vi "Begin.vi"(11 "Image Size":T1=enum."320x240") -> (0 "error out":errorcluster)   [LabVIEW 2012]
doc: "Called before other user functions, this VI is expected to open initial I/O refnums, load in file data, and do all program initialization. Notice that the <B>error out</B> terminal is simply used for data flow. Wiring it to other structures or subVIs ensures that this VI runs first."
uses:
  <vilib>/Rock Robotics/WPI/Camera/WPI_CameraImageSize.ctl
  <vilib>/Rock Robotics/WPI/DriverStation/WPI_DriverStationRobotMode2.ctl
  <vilib>/Rock Robotics/SystemInterfaces/DIO/FPGA_DIOPWMChannel.ctl
  <vilib>/Rock Robotics/WPI/Joystick/WPI_JoystickDeviceEnum.ctl
  <vilib>/Rock Robotics/WPI/Relay/WPI_RelayDirection.ctl
  <vilib>/Rock Robotics/SystemInterfaces/DIO/FPGA_DIORelayChannel.ctl
  <vilib>/Rock Robotics/SystemInterfaces/AI/FPGA_AIChannel.ctl
  <vilib>/Rock Robotics/SystemInterfaces/AI/FPGA_AIGyroChannel.ctl
  <vilib>/Rock Robotics/SystemInterfaces/DIO/FPGA_DIOChannel.ctl
  <vilib>/Rock Robotics/SystemInterfaces/Typedef/FPGA_TypedefDigitalModule.ctl
  Robot Global Data.vi
  <vilib>/Rock Robotics/WPI/MotorControl/WPI_MotorControlOpen Victor.vi
  <vilib>/Rock Robotics/WPI/Camera/WPI_CameraFrameRate.ctl
panel:
  in  "Input":dbl
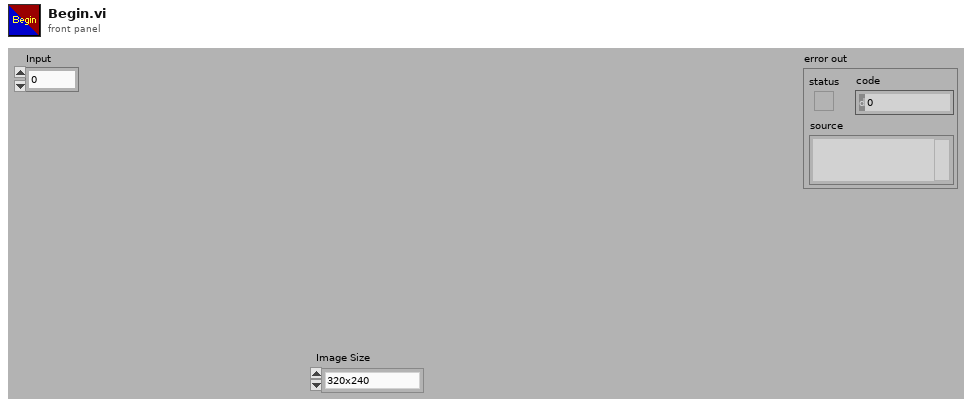
[diagram p1: front panel]
types:
  T1 = typedef "WPI_CameraImageSize.ctl" = enum16{"640x480", "320x240", "160x120"}
  T2 = typedef "FPGA_DIOChannel.ctl" = enum8{"DIO 1", "DIO 2", "DIO 3", "DIO 4", "DIO 5", "DIO 6", "DIO 7", "DIO 8", "DIO 9", "DIO 10", "DIO 11", "DIO 12", "DIO 13", "DIO 14", "Invalid"}
  T3 = typedef "FPGA_TypedefDigitalModule.ctl" = enum16{"Digital Module 1", "Digital Module 2"}
  T4 = typedef "FPGA_DIOPWMChannel.ctl" = enum8{"PWM 1", "PWM 2", "PWM 3", "PWM 4", "PWM 5", "PWM 6", "PWM 7", "PWM 8", "PWM 9", "PWM 10", "Invalid"}
  T5 = typedef "FPGA_DIORelayChannel.ctl" = enum8{"Relay 1", "Relay 2", "Relay 3", "Relay 4", "Relay 5", "Relay 6", "Relay 7", "Relay 8", "Invalid"}
  T6 = typedef "WPI_RelayDirection.ctl" = enum16{"Both directions", "Forward only", "Reverse only"}
  T7 = typedef "FPGA_AIChannel.ctl" = enum8{"AI 1", "AI 2", "AI 3", "AI 4", "AI 5", "AI 6", "AI 7", "AI 8", "Invalid"}
  T8 = typedef "FPGA_AIGyroChannel.ctl" = enum8{"AI 1", "AI 2", "Invalid"}
  T9 = typedef "WPI_JoystickDeviceEnum.ctl" = enum16{"USB 1", "USB 2", "USB 3", "USB 4", "Kinect 1", "Kinect 2"}
  T10 = typedef "WPI_DriverStationRobotMode2.ctl" = enum16{"Autonomous Disabled", "Autonomous Enabled", "Teleop Disabled", "Teleop Enabled", "Timeout", "Finish", "Test Disabled", "Test Enabled"}
  T11 = typedef "WPI_RelayDevRef.ctl" = cluster{"DevStatus":errorcluster, "Relay Channel":T5, "Digital Module":T3, "Relay Direction":T6}
  T12 = typedef "WPI_CameraFrameRate.ctl" = u32
  T13 = typedef "WPI_CameraDevRef.ctl" = cluster{"Camera Address":string, "CameraStatus":errorcluster, "Acquire Image Notifier":refnum<notifier>}
  T14 = typedef "WPI_MotorControlDeviceRef.ctl" = cluster{"DeviceStatus":errorcluster, "Type":enum16{"PWM", "CAN"}, "PWM":cluster{"Digital Module":T3, "PWM Channel":T4, "DeadBand":T15}, "CAN":cluster{"Device Number":u8, "Control Mode":T16, "Semaphore":T17, "Max Vout":dbl}, "Invert":bool, "TransformRef":T18, "InvTransformRef":T18}
  T15 = typedef "WPI_PWMDeadband.ctl" = cluster{"Name":string, "maxPositivePwm":i32, "minPositivePwm":i32, "centerPwm":i32, "maxNegativePwm":i32, "minNegativePwm":i32, "angularRange":u16}
  T16 = typedef "WPI_CANJaguar_ControlMode.ctl" = enum8{"Percent VBus", "Current", "Speed", "Position", "Voltage"}
  T17 = typedef "Semaphore RefNum" = refnum<k1>
  T18 = typedef "WPI_PWMTransform_ConPane.ctl" = refnum<vi>
  T19 = typedef "WPI_JoystickDevRef.ctl" = cluster{"Device":T9}
  T20 = typedef "WPI_ServoDeviceRef.ctl" = cluster{"DeviceStatus":errorcluster, "Digital Module":T3, "PWM Channel":T4, "DeadBand":T15}
  T21 = cluster{"Setpoint 1":dbl, "Setpoint 2":dbl, "Setpoint 3":dbl, "Setpoint 4":dbl, "RotLow":dbl, "RotHigh":dbl, "ExtLow":dbl, "ExtHigh":dbl}
  T22 = typedef "WPI_DigitalInputDevRef.ctl" = cluster{"DevStatus":errorcluster, "DIO Channel":T2, "Digital Module":T3}
  T23 = typedef "WPI_AnalogChannelDevRef.ctl" = cluster{"DevStatus":errorcluster, "Analog Module":T24, "Analog Channel":T7}
  T24 = typedef "FPGA_TypedefAnalogModule.ctl" = enum16{"Analog Module 1", "Analog Module 2"}
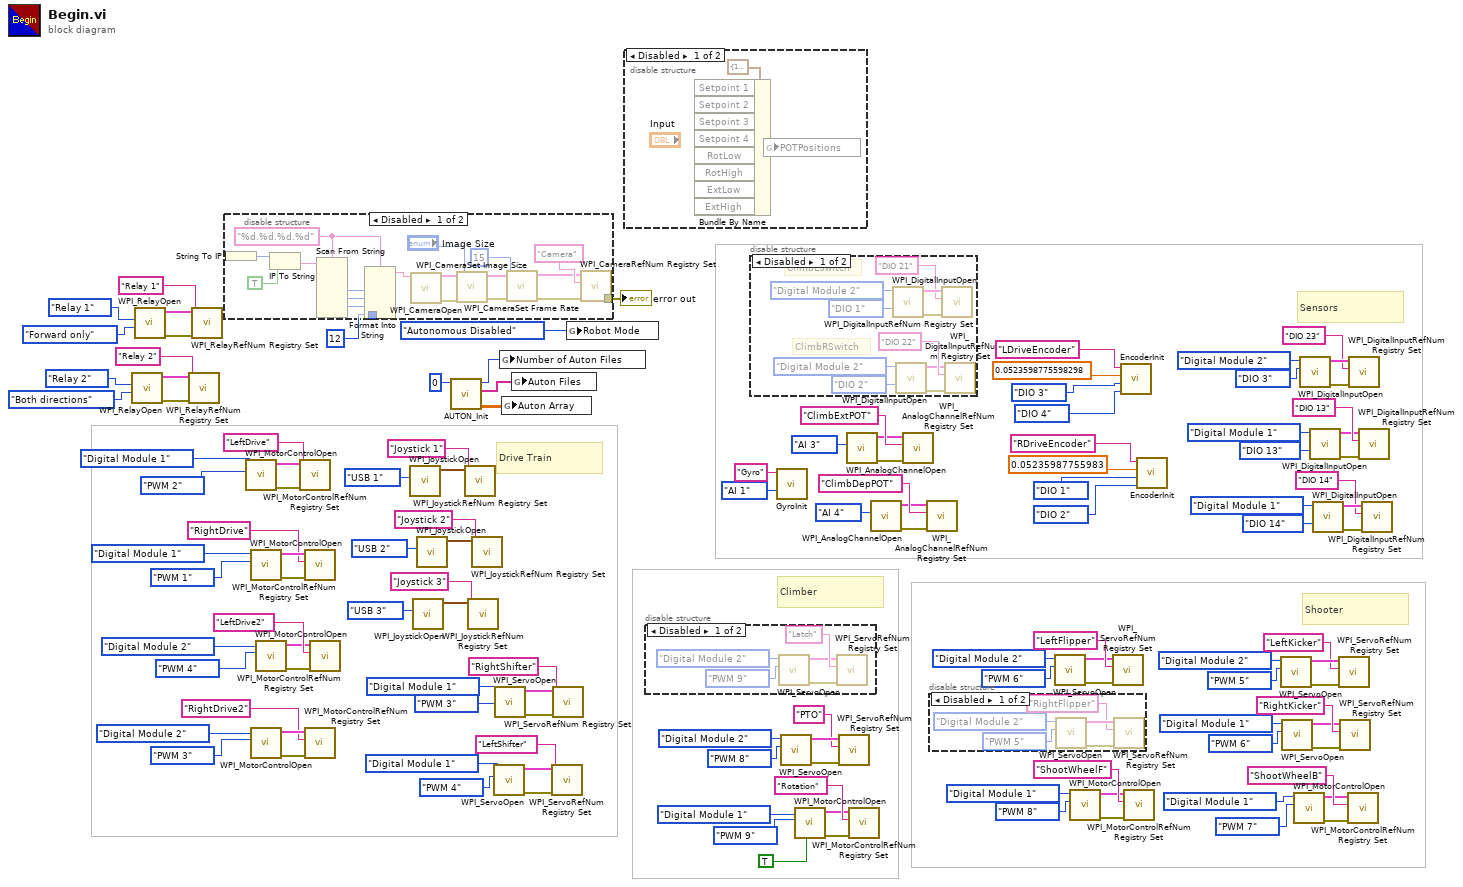
[diagram p0: block diagram]
diagram:
  # "Shooter"
  # "Drive Train"
  # "Climber"
  # "Sensors"
  n1 = call <vilib>:"WPI_RelayOpen.vi"("Relay Direction"=WPI_RelayDirection."Both directions", "Relay Channel"=FPGA_DIORelayChannel."Relay 2") -> ("error out"=w87:errorcluster, "RelayDevRef"=w88:T11)  [unwired: 8 in]
  n2 = call <vilib>:"WPI_RelayOpen.vi"("Relay Direction"=WPI_RelayDirection."Forward only", "Relay Channel"=FPGA_DIORelayChannel."Relay 1") -> ("error out"=w45:errorcluster, "RelayDevRef"=w44:T11)  [unwired: 8 in]
  n3 = call <vilib>:"WPI_RelayRefNum Registry Set.vi"("error in (no error)"=w87, "refnum name"="Relay 2", "RelayDevRef"=w88) -> ()  [unwired: 7 in, 2 out]
  n4 = call <vilib>:"WPI_RelayRefNum Registry Set.vi"("error in (no error)"=w45, "refnum name"="Relay 1", "RelayDevRef"=w44) -> ()  [unwired: 7 in, 2 out]
  n5 = disable-structure shown="Disabled" {
    disable-tunnel: 12 ("Compression") -> [w136 _]
    disable-tunnel: [w126 _] -> w46
    frame Disabled {
      w135 = "%d.%d.%d.%d" ("format string")
      n6 = String To IP() -> (0:w142:u32)  [unwired: 1 in]
      n7 = IP To String(1:TRUE ("dot notation? (F)"), 2:w142) -> (0:w140:string)
      n8 = Scan From String(format string=w135, input string=w140) -> (output 1=w139:i32, output 2=w138:i32, output 3=w137:i32)  [unwired: 7 in, 3 out]
      n9 = Format Into String(format string=w135, w139, w138, w137, w136) -> (resulting string=w134:string)  [unwired: 2 in, 1 out]
      n10 = call <vilib>:"WPI_CameraOpen.vi"("Camera Address"=w134) -> ("error out"=w133:errorcluster, "CameraDevRef"=w132:T13)  [unwired: 1 in, 8 out]
      n11 = call <vilib>:"WPI_CameraSet Image Size.vi"("error in (no error)"=w133, "Image Size"="Image Size", "CameraDevRef"=w132) -> ("error out"=w130:errorcluster, "CameraDevRef Out"=w131:T13)  [unwired: 7 out]
      n12 = call <vilib>:"WPI_CameraSet Frame Rate.vi"("error in (no error)"=w130, "Frame Rate (fps)"=T12 15, "CameraDevRef"=w131) -> ("error out"=w129:errorcluster, "CameraDevRef Out"=w128:T13)  [unwired: 7 out]
      n13 = call <vilib>:"WPI_CameraRefNum Registry Set.vi"("error in (no error)"=w129, "refnum name"="Camera", "CameraDevRef"=w128) -> ("error out"=w126:errorcluster)  [unwired: 8 out]
    }
    frame Enabled {
    }
  }
  "error out" <- w46
  n14 = call-poly <vilib>:"WPI_MotorControlOpen.vi"("PWM Channel"=FPGA_DIOPWMChannel."PWM 2", "Digital Module (Module 1)"=FPGA_TypedefDigitalModule."Digital Module 1") -> ("error out"=w113:errorcluster, "MotorControlDeviceRef"=w114:T14)  [unwired: 8 in]
  n15 = call-poly <vilib>:"WPI_MotorControlOpen.vi"("PWM Channel"=FPGA_DIOPWMChannel."PWM 1", "Digital Module (Module 1)"=FPGA_TypedefDigitalModule."Digital Module 1") -> ("error out"=w120:errorcluster, "MotorControlDeviceRef"=w119:T14)  [unwired: 8 in]
  n16 = call-poly <vilib>:"WPI_MotorControlOpen.vi"("PWM Channel"=FPGA_DIOPWMChannel."PWM 3", "Digital Module (Module 1)"=FPGA_TypedefDigitalModule."Digital Module 2") -> ("error out"=w102:errorcluster, "MotorControlDeviceRef"=w101:T14)  [unwired: 8 in]
  n17 = call-poly <vilib>:"WPI_MotorControlOpen.vi"("PWM Channel"=FPGA_DIOPWMChannel."PWM 4", "Digital Module (Module 1)"=FPGA_TypedefDigitalModule."Digital Module 2") -> ("error out"=w93:errorcluster, "MotorControlDeviceRef"=w94:T14)  [unwired: 8 in]
  n18 = call <vilib>:"WPI_MotorControlRefNum Registry Set.vi"("error in (no error)"=w113, "refnum name"="LeftDrive", "MotorControlDevRef"=w114) -> ()  [unwired: 7 in, 2 out]
  n19 = call <vilib>:"WPI_MotorControlRefNum Registry Set.vi"("error in (no error)"=w120, "refnum name"="RightDrive", "MotorControlDevRef"=w119) -> ()  [unwired: 7 in, 2 out]
  n20 = call <vilib>:"WPI_MotorControlRefNum Registry Set.vi"("error in (no error)"=w102, "refnum name"="RightDrive2", "MotorControlDevRef"=w101) -> ()  [unwired: 7 in, 2 out]
  n21 = call <vilib>:"WPI_MotorControlRefNum Registry Set.vi"("error in (no error)"=w93, "refnum name"="LeftDrive2", "MotorControlDevRef"=w94) -> ()  [unwired: 7 in, 2 out]
  n22 = call <vilib>:"WPI_JoystickOpen.vi"("JoystickDevice"=WPI_JoystickDeviceEnum."USB 1") -> ("JoystickDevRef"=w104:T19)  [unwired: 10 in]
  n23 = call <vilib>:"WPI_JoystickOpen.vi"("JoystickDevice"=WPI_JoystickDeviceEnum."USB 3") -> ("JoystickDevRef"=w110:T19)  [unwired: 10 in]
  n24 = call <vilib>:"WPI_JoystickOpen.vi"("JoystickDevice"=WPI_JoystickDeviceEnum."USB 2") -> ("JoystickDevRef"=w109:T19)  [unwired: 10 in]
  n25 = call "AUTON_Init.vi"("Default File"=0) -> ("Auton Array"=w121:dbl[][], "Auton Files"=w122:string[], "Number of Auton Files"=w123:i64)  [unwired: 8 in]
  n26 = call <vilib>:"WPI_JoystickRefNum Registry Set.vi"("refnum name"="Joystick 1", "JoystickDevRef"=w104) -> ()  [unwired: 8 in, 2 out]
  n27 = call <vilib>:"WPI_JoystickRefNum Registry Set.vi"("refnum name"="Joystick 3", "JoystickDevRef"=w110) -> ()  [unwired: 8 in, 2 out]
  n28 = call <vilib>:"WPI_JoystickRefNum Registry Set.vi"("refnum name"="Joystick 2", "JoystickDevRef"=w109) -> ()  [unwired: 8 in, 2 out]
  n29 = call <vilib>:"WPI_ServoOpen.vi"("PWM Channel"=FPGA_DIOPWMChannel."PWM 4", "Digital Module (Module 1)"=FPGA_TypedefDigitalModule."Digital Module 1") -> ("error out"=w86:errorcluster, "ServoDeviceRef"=w79:T20)  [unwired: 8 in]
  n30 = call <vilib>:"WPI_ServoOpen.vi"("PWM Channel"=FPGA_DIOPWMChannel."PWM 3", "Digital Module (Module 1)"=FPGA_TypedefDigitalModule."Digital Module 1") -> ("error out"=w85:errorcluster, "ServoDeviceRef"=w84:T20)  [unwired: 8 in]
  n31 = global write "Robot Global Data.vi" "Number of Auton Files"(w123) -> ()
  n32 = global write "Robot Global Data.vi" "Auton Array"(w121) -> ()
  n33 = global write "Robot Global Data.vi" "Auton Files"(w122) -> ()
  n34 = call <vilib>:"WPI_ServoRefNum Registry Set.vi"("error in (no error)"=w86, "refnum name"="LeftShifter", "ServoDeviceRef"=w79) -> ()  [unwired: 7 in, 2 out]
  n35 = call <vilib>:"WPI_ServoRefNum Registry Set.vi"("error in (no error)"=w85, "refnum name"="RightShifter", "ServoDeviceRef"=w84) -> ()  [unwired: 7 in, 2 out]
  n36 = global write "Robot Global Data.vi" "Robot Mode"(WPI_DriverStationRobotMode2."Autonomous Disabled" ("Robot Mode")) -> ()
  n37 = disable-structure shown="Disabled" {
    frame Disabled {
      n38 = Bundle By Name(cluster=T21 {"Setpoint 1"=1.95, "Setpoint 2"=2.1, "Setpoint 3"=2.2, "Setpoint 4"=2.25, "RotLow"=1.92, "RotHigh"=2.3, "ExtLow"=1.87, "ExtHigh"=1.97} ("POTPositions")) -> (w145:T21)  [unwired: 8 in]
      n39 = global write "Robot Global Data.vi" "POTPositions"(w145) -> ()
    }
    frame Enabled {
    }
  }
  n40 = disable-structure shown="Disabled" {
    frame Disabled {
      n41 = call <vilib>:"WPI_ServoOpen.vi"("PWM Channel"=FPGA_DIOPWMChannel."PWM 9", "Digital Module (Module 1)"=FPGA_TypedefDigitalModule."Digital Module 2") -> ("error out"=w148:errorcluster, "ServoDeviceRef"=w149:T20)  [unwired: 8 in]
      n42 = call <vilib>:"WPI_ServoRefNum Registry Set.vi"("error in (no error)"=w148, "refnum name"="Latch", "ServoDeviceRef"=w149) -> ()  [unwired: 7 in, 2 out]
    }
    frame Enabled {
    }
  }
  n43 = disable-structure shown="Disabled" {
    frame Disabled {
      # "ClimbRSwitch"
      # "ClimbLSwitch"
      n44 = call <vilib>:"WPI_DigitalInputOpen.vi"("DIO Channel"=FPGA_DIOChannel."DIO 1", "Digital Module (Module 1)"=FPGA_TypedefDigitalModule."Digital Module 2") -> ("error out"=w153:errorcluster, "DigitalInputDevRef"=w154:T22)  [unwired: 8 in]
      n45 = call <vilib>:"WPI_DigitalInputOpen.vi"("DIO Channel"=FPGA_DIOChannel."DIO 2", "Digital Module (Module 1)"=FPGA_TypedefDigitalModule."Digital Module 2") -> ("error out"=w160:errorcluster, "DigitalInputDevRef"=w159:T22)  [unwired: 8 in]
      n46 = call <vilib>:"WPI_DigitalInputRefNum Registry Set.vi"("error in (no error)"=w153, "refnum name"="DIO 21", "DigitalInputDevRef"=w154) -> ()  [unwired: 7 in, 2 out]
      n47 = call <vilib>:"WPI_DigitalInputRefNum Registry Set.vi"("error in (no error)"=w160, "refnum name"="DIO 22", "DigitalInputDevRef"=w159) -> ()  [unwired: 7 in, 2 out]
    }
    frame Enabled {
    }
  }
  n48 = call "GyroInit.vi"("refnum name"="Gyro", "Analog Channel"=FPGA_AIGyroChannel."AI 1") -> ()  [unwired: 8 in]
  n49 = call <vilib>:"WPI_ServoOpen.vi"("PWM Channel"=FPGA_DIOPWMChannel."PWM 8", "Digital Module (Module 1)"=FPGA_TypedefDigitalModule."Digital Module 2") -> ("error out"=w64:errorcluster, "ServoDeviceRef"=w63:T20)  [unwired: 8 in]
  n50 = call-poly <vilib>:"WPI_MotorControlOpen.vi"("Invert"=TRUE, "PWM Channel"=FPGA_DIOPWMChannel."PWM 9", "Digital Module (Module 1)"=FPGA_TypedefDigitalModule."Digital Module 1") -> ("error out"=w69:errorcluster, "MotorControlDeviceRef"=w68:T14)  [unwired: 7 in]
  n51 = call <vilib>:"WPI_ServoRefNum Registry Set.vi"("error in (no error)"=w64, "refnum name"="PTO", "ServoDeviceRef"=w63) -> ()  [unwired: 7 in, 2 out]
  n52 = call <vilib>:"WPI_AnalogChannelOpen.vi"("Analog Channel"=FPGA_AIChannel."AI 3") -> ("error out"=w48:errorcluster, "AIDeviceRef"=w49:T23)  [unwired: 9 in]
  n53 = call <vilib>:"WPI_MotorControlRefNum Registry Set.vi"("error in (no error)"=w69, "refnum name"="Rotation", "MotorControlDevRef"=w68) -> ()  [unwired: 7 in, 2 out]
  n54 = call <vilib>:"WPI_AnalogChannelOpen.vi"("Analog Channel"=FPGA_AIChannel."AI 4") -> ("error out"=w73:errorcluster, "AIDeviceRef"=w74:T23)  [unwired: 9 in]
  n55 = call <vilib>:"WPI_AnalogChannelRefNum Registry Set.vi"("error in (no error)"=w48, "refnum name"="ClimbExtPOT", "AIDeviceRef"=w49) -> ()  [unwired: 7 in, 2 out]
  n56 = call <vilib>:"WPI_AnalogChannelRefNum Registry Set.vi"("error in (no error)"=w73, "refnum name"="ClimbDepPOT", "AIDeviceRef"=w74) -> ()  [unwired: 7 in, 2 out]
  n57 = disable-structure shown="Disabled" {
    frame Disabled {
      n58 = call <vilib>:"WPI_ServoOpen.vi"("PWM Channel"=FPGA_DIOPWMChannel."PWM 5", "Digital Module (Module 1)"=FPGA_TypedefDigitalModule."Digital Module 2") -> ("error out"=w166:errorcluster, "ServoDeviceRef"=w165:T20)  [unwired: 8 in]
      n59 = call <vilib>:"WPI_ServoRefNum Registry Set.vi"("error in (no error)"=w166, "refnum name"="RightFlipper", "ServoDeviceRef"=w165) -> ()  [unwired: 7 in, 2 out]
    }
    frame Enabled {
    }
  }
  n60 = call <vilib>:"WPI_ServoOpen.vi"("PWM Channel"=FPGA_DIOPWMChannel."PWM 6", "Digital Module (Module 1)"=FPGA_TypedefDigitalModule."Digital Module 2") -> ("error out"=w26:errorcluster, "ServoDeviceRef"=w27:T20)  [unwired: 8 in]
  n61 = call-poly <vilib>:"WPI_MotorControlOpen.vi"("PWM Channel"=FPGA_DIOPWMChannel."PWM 8", "Digital Module (Module 1)"=FPGA_TypedefDigitalModule."Digital Module 1") -> ("error out"=w37:errorcluster, "MotorControlDeviceRef"=w38:T14)  [unwired: 8 in]
  n62 = call <vilib>:"WPI_ServoRefNum Registry Set.vi"("error in (no error)"=w26, "refnum name"="LeftFlipper", "ServoDeviceRef"=w27) -> ()  [unwired: 7 in, 2 out]
  n63 = call "EncoderInit.vi"("refnum name"="LDriveEncoder", "DistancePerCount"=0.0523598775598298, "DIO Channel"=FPGA_DIOChannel."DIO 3", "DIO Channel 2"=FPGA_DIOChannel."DIO 4") -> ()  [unwired: 7 in]
  n64 = call <vilib>:"WPI_MotorControlRefNum Registry Set.vi"("error in (no error)"=w37, "refnum name"="ShootWheelF", "MotorControlDevRef"=w38) -> ()  [unwired: 7 in, 2 out]
  n65 = call "EncoderInit.vi"("refnum name"="RDriveEncoder", "DistancePerCount"=0.05235987755983, "DIO Channel"=FPGA_DIOChannel."DIO 1", "DIO Channel 2"=FPGA_DIOChannel."DIO 2") -> ()  [unwired: 7 in]
  n66 = call <vilib>:"WPI_ServoOpen.vi"("PWM Channel"=FPGA_DIOPWMChannel."PWM 5", "Digital Module (Module 1)"=FPGA_TypedefDigitalModule."Digital Module 2") -> ("error out"=w21:errorcluster, "ServoDeviceRef"=w20:T20)  [unwired: 8 in]
  n67 = call <vilib>:"WPI_ServoOpen.vi"("PWM Channel"=FPGA_DIOPWMChannel."PWM 6", "Digital Module (Module 1)"=FPGA_TypedefDigitalModule."Digital Module 1") -> ("error out"=w16:errorcluster, "ServoDeviceRef"=w22:T20)  [unwired: 8 in]
  n68 = call-poly <vilib>:"WPI_MotorControlOpen.vi"("PWM Channel"=FPGA_DIOPWMChannel."PWM 7", "Digital Module (Module 1)"=FPGA_TypedefDigitalModule."Digital Module 1") -> ("error out"=w33:errorcluster, "MotorControlDeviceRef"=w32:T14)  [unwired: 8 in]
  n69 = call <vilib>:"WPI_DigitalInputOpen.vi"("DIO Channel"=FPGA_DIOChannel."DIO 3", "Digital Module (Module 1)"=FPGA_TypedefDigitalModule."Digital Module 2") -> ("error out"=w1:errorcluster, "DigitalInputDevRef"=w4:T22)  [unwired: 8 in]
  n70 = call <vilib>:"WPI_DigitalInputOpen.vi"("DIO Channel"=FPGA_DIOChannel."DIO 13", "Digital Module (Module 1)"=FPGA_TypedefDigitalModule."Digital Module 1") -> ("error out"=w14:errorcluster, "DigitalInputDevRef"=w13:T22)  [unwired: 8 in]
  n71 = call <vilib>:"WPI_DigitalInputOpen.vi"("DIO Channel"=FPGA_DIOChannel."DIO 14", "Digital Module (Module 1)"=FPGA_TypedefDigitalModule."Digital Module 1") -> ("error out"=w7:errorcluster, "DigitalInputDevRef"=w8:T22)  [unwired: 8 in]
  n72 = call <vilib>:"WPI_ServoRefNum Registry Set.vi"("error in (no error)"=w21, "refnum name"="LeftKicker", "ServoDeviceRef"=w20) -> ()  [unwired: 7 in, 2 out]
  n73 = call <vilib>:"WPI_ServoRefNum Registry Set.vi"("error in (no error)"=w16, "refnum name"="RightKicker", "ServoDeviceRef"=w22) -> ()  [unwired: 7 in, 2 out]
  n74 = call <vilib>:"WPI_MotorControlRefNum Registry Set.vi"("error in (no error)"=w33, "refnum name"="ShootWheelB", "MotorControlDevRef"=w32) -> ()  [unwired: 7 in, 2 out]
  n75 = call <vilib>:"WPI_DigitalInputRefNum Registry Set.vi"("error in (no error)"=w1, "refnum name"="DIO 23", "DigitalInputDevRef"=w4) -> ()  [unwired: 7 in, 2 out]
  n76 = call <vilib>:"WPI_DigitalInputRefNum Registry Set.vi"("error in (no error)"=w14, "refnum name"="DIO 13", "DigitalInputDevRef"=w13) -> ()  [unwired: 7 in, 2 out]
  n77 = call <vilib>:"WPI_DigitalInputRefNum Registry Set.vi"("error in (no error)"=w7, "refnum name"="DIO 14", "DigitalInputDevRef"=w8) -> ()  [unwired: 7 in, 2 out]
